vi "Initialize.vi"(6 "timeout in ms":i32=30000, 7 "Engine Configuration":refnum<class "engine configuration.lvclass">, 8 "error in":errorcluster, 9 "Module Configurations":refnum<class "TBM module configuration.lvclass">[](array[class]), 10 "Modules":refnum<class "TBM module execution interface.lvclass">[](array[class]), 11 "Standard Engine in":refnum<class "Standard Engine Runtime.lvclass">) -> (0 "error out":errorcluster, 3 "Standard Engine out":refnum<class "Standard Engine Runtime.lvclass">)   [LabVIEW 2013, in "Standard Engine Runtime.lvclass"]
uses:
  Standard Engine Runtime.lvclass
  <vilib>/NI/Tag Bus Module Framework/module configuration/TBM module configuration.lvclass
  <vilib>/NI/Tag Bus Module Framework/runtime/TBM module execution interface.lvclass
  <vilib>/NI/Module Execution Interface/Engine Configuration/engine configuration.lvclass
  Commands.ctl
  Configuration/Standard Engine Configuration.lvclass
  Engine Config Data.ctl
  <vilib>/NI/Module Execution Interface/Engine Runtime/Execution States.ctl
  Standard Engine Runtime.lvclass/Standard Engine Runtime.ctl
  <vilib>/NI/Module Execution Interface/Engine Runtime/Engine Runtime Interface.lvclass
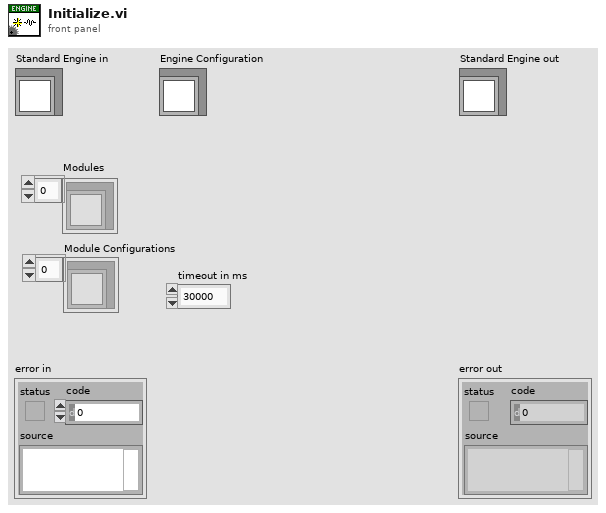
[diagram p1: front panel]
types:
  T1 = typedef "Engine Runtime Interface.lvclass/Execution States.ctl" = enum16{"Initializing", "Paused (Initialized)", "Running", "Set Safe Outputs", "Uninitializing", "Stopped (Uninitialized)", "Error (Uninitialized)", "Safe State (Uninitialized)", "Closed"}
  T2 = typedef "Standard Engine Runtime.lvclass/Engine Config Data.ctl" = cluster{"Engine Configuration":refnum<class "Standard Engine Configuration.lvclass">, "Modules":refnum<class "TBM module execution interface.lvclass">[], "Module Configurations":refnum<class "TBM module configuration.lvclass">[]}
  T3 = typedef "Standard Engine Runtime.lvclass/Commands.ctl" = enum16{"Initialize", "Start", "Pause", "Safe State", "Normal", "Stop", "Shutdown"}
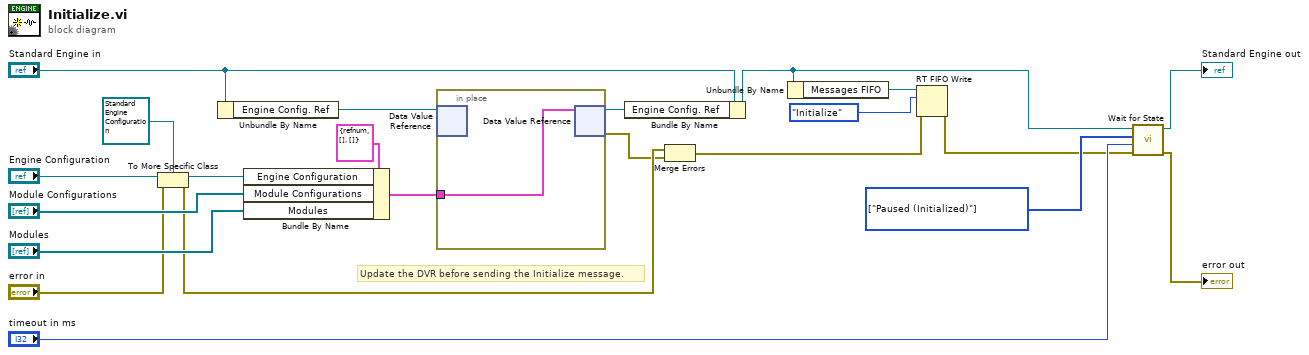
[diagram p0: block diagram]
diagram:
  w5 = T1[] [enum."Paused (Initialized)"] items=["Initializing", "Paused (Initialized)", "Running", "Set Safe Outputs", "Uninitializing", "Stopped (Uninitialized)", "Error (Uninitialized)", "Safe State (Uninitialized)", "Closed"] ("expected states")
  # "Update the DVR before sending the Initialize message."
  n1 = To More Specific Class(target class=refnum<class "Standard Engine Configuration.lvclass"> refnum ("Engine Configuration"), reference="Engine Configuration", error in="error in") -> (specific class reference=w16:refnum<class "Standard Engine Configuration.lvclass">, error out=w9:errorcluster)
  n2 = Unbundle By Name("Standard Engine in") -> ("Engine Config. Ref"=w12:refnum<data-value>)
  n3 = Bundle By Name(cluster=T2 {"Engine Configuration"=refnum, "Modules"=[], "Module Configurations"=[]} ("Engine Configuration Data"), "Engine Configuration"=w16, "Module Configurations"="Module Configurations", "Modules"="Modules") -> (w10:T2)
  n4 = in-place {
    in-place-border: w10 -> [w23]
    n5 = in-place-dvr #1(w12) -> ()  [unwired: 2 out]
    n6 = in-place-dvr #1(w23) -> (w11:refnum<data-value>, w8:errorcluster)
  }
  n7 = Bundle By Name(cluster="Standard Engine in", "Engine Config. Ref"=w11) -> (w2:refnum<class "Standard Engine Runtime.lvclass">)
  n8 = Merge Errors(w9, w8) -> (w7:errorcluster)
  n9 = Unbundle By Name(w2) -> ("Messages FIFO"=w22:refnum<k33>)
  n10 = RT FIFO Write(0:w22, 1:Commands."Initialize" ("element"), 3:w7) -> (11:w4:errorcluster)  [unwired: 2 in, 3 out]
  n11 = call "Wait for State.vi"("error in"=w4, "timeout in ms"="timeout in ms", "expected states"=w5, "Standard Engine in"=w2) -> ("error out"=→"error out":errorcluster, "Standard Engine out"=→"Standard Engine out":refnum<class "Standard Engine Runtime.lvclass">)  [unwired: 6 in]
